vi "Var to Boolean 2D.vi"(11 "Variant":variant) -> (3 "Bool 2D":bool[][](array[boolean]))   [LabVIEW 2016]
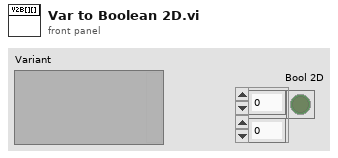
[diagram p1: front panel]
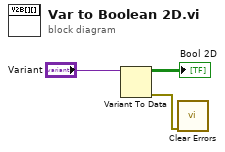
[diagram p0: block diagram]
diagram:
  n1 = Variant To Data(Variant="Variant") -> (data=→"Bool 2D":bool[][], error out=w2:errorcluster)  [unwired: 2 in]
  n2 = call <vilib>:"Clear Errors.vi"("error in (no error)"=w2) -> ()  [unwired: 5 in, 2 out]
